vi "Record_CreateAvi.vi"(8 "error in":errorcluster, 10 "Settings in":T4={"Harware Configuration"={"Camera"="cam1", "Frames Per Second"=15, "Simulate Recording"=FALSE, "Simulated Recording Sample"=path "", "Timestamp Method"=enum."Camera Timestamp"}, "Base Recording Path"=path "", "Type Of Recording"="", "Recording Codec"="", "TrackingSettings"={"Max Radius"=0, "Threshold"=160.0, "ROI"={"Left"=0, "Top"=0, "Right"=0, "Bottom"=0, "Rotation"=0.0}}, "Calibration"={"Pixel Width (X)"=1.0, "Pixel Height (Y)"=1.0}, "Broadcast Length"=0} {"Broadcast Length" min=0; "TrackingSettings"."ROI"."Rotation" format="%.2f"; "TrackingSettings"."ROI"."Left" scale=0.0..1024.0; "TrackingSettings"."ROI"."Right" scale=0.0..1024.0; "TrackingSettings"."Threshold" scale=0.0..255.0}, 11 "Recording Data In":T1) -> (0 "error out":errorcluster, 3 "Recording Data Out":T1)   [LabVIEW 2017, in "ImageAcquisitionLibrary.lvlib"]
uses:
  ImageAcquisitionLibrary.lvlib
  Settings/Settings.ctl
  <vilib>/userdefined/High Color/IMAQdx.ctl
  Tracking/TrackingSettings.ctl
  Settings/Calibration.ctl
  RecordingData.ctl
  <vilib>/vision/Image Controls.llb/IMAQ Image.ctl
  <vilib>/vision/Avi.llb/IMAQ AVI2 Refnum.ctl
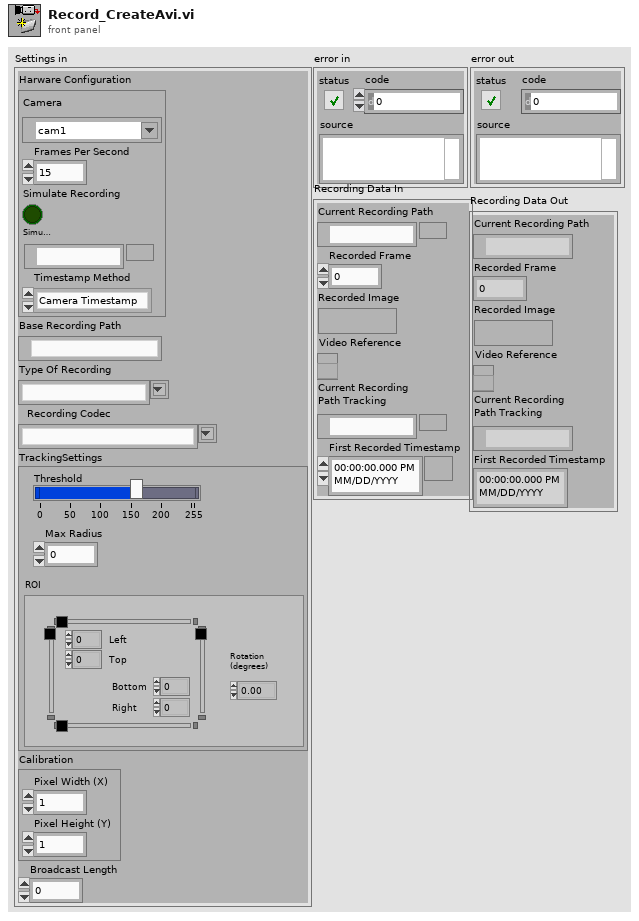
[diagram p1: front panel]
types:
  T1 = typedef "ImageAcquisitionLibrary.lvlib/RecordingData.ctl" = cluster{"Current Recording Path":path, "Recorded Frame":i32, "Recorded Image":T2, "Video Reference":T3, "Current Recording \nPath Tracking":path, "First Recorded Timestamp":timestamp}
  T2 = typedef "IMAQ Image.ctl" = refnum<image>
  T3 = typedef "IMAQ AVI2 Refnum.ctl" = refnum<k20>
  T4 = typedef "ImageAcquisitionLibrary.lvlib/Settings.ctl" = cluster{"Harware Configuration":cluster{"Camera":T5, "Frames Per Second":u32, "Simulate Recording":bool, "Simulated Recording Sample":path, "Timestamp Method":enum16{"System Timestamp", "Camera Timestamp", "IMAQdx Timestamp"}}, "Base Recording Path":path, "Type Of Recording":string, "Recording Codec":string, "TrackingSettings":T6, "Calibration":T8, "Broadcast Length":i32}
  T5 = typedef "IMAQdx.ctl" = refnum<k21>
  T6 = typedef "ImageAcquisitionLibrary.lvlib/TrackingSettings.ctl" = cluster{"Max Radius":i32, "Threshold":sgl, "ROI":T7}
  T7 = typedef "IMAQ Rectangle" = cluster{"Left":i32, "Top":i32, "Right":i32, "Bottom":i32, "Rotation":dbl}
  T8 = typedef "ImageAcquisitionLibrary.lvlib/Calibration.ctl" = cluster{"Pixel Width (X)":dbl, "Pixel Height (Y)":dbl}
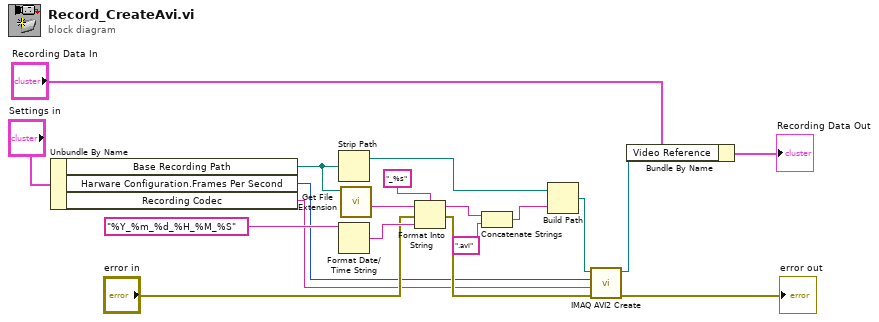
[diagram p0: block diagram]
diagram:
  n1 = Unbundle By Name("Settings in") -> ("Base Recording Path"=w12:path, "Harware Configuration.Frames Per Second"=w6:u32, "Recording Codec"=w7:string)
  n2 = Strip Path(path=w12) -> (stripped path=w18:path)  [unwired: 1 out]
  n3 = Format Date/Time String(time format string (%c)="%Y_%m_%d_%H_%M_%S") -> (date/time string=w16:string)  [unwired: 2 in]
  n4 = call <vilib>:"Get File Extension.vi"("file"=w12) -> ("filename without extension"=w19:string)  [unwired: 6 in, 4 out]
  n5 = Format Into String(format string="_%s", initial string=w19, error in="error in", w16) -> (resulting string=w3:string, error out=w10:errorcluster)
  n6 = Concatenate Strings(w3, ".avi" ("string")) -> (w2:string)
  n7 = Build Path(base path=w18, name or relative path=w2) -> (appended path=w11:path)
  n8 = call "IMAQ AVI2 Create"("error in (no error)"=w10, "Codec"=w7, "Frames Per Second"=w6, "AVI Path"=w11) -> ("error out"=→"error out":errorcluster, "AVI Refnum"=w8:T3)  [unwired: 6 in]
  n9 = Bundle By Name(cluster="Recording Data In", "Video Reference"=w8) -> (→"Recording Data Out":T1)
